vi "libdaq_counter_config.vi"(0 "error in (no error)":errorcluster, 1 "device_name":string, 2 "module_name":string, 3 "mode":T2(ring), 4 "edge":T1(ring), 5 "period":i32) -> (14 "error out":errorcluster, 15 "device_name":string, 16 "module_name":string)   [LabVIEW 2010, in "libdaqVI.lvlib"]
uses:
  libdaqVI.lvlib
  dll/daqlib.dll
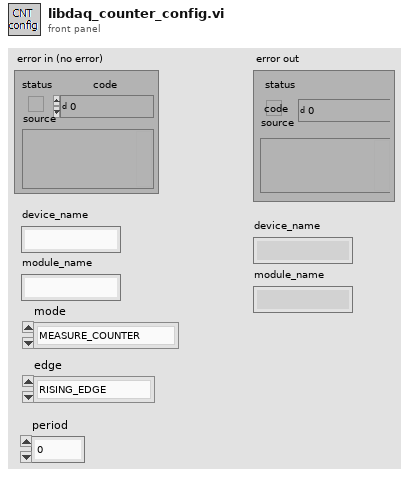
[diagram p1: front panel]
types:
  T1 = enum16{"RISING_EDGE", "FALLING_EDGE", "BOTH_EDGE"}
  T2 = enum16{"MEASURE_COUNTER", "MEASURE_PERIOD", "MEASURE_PWM"}
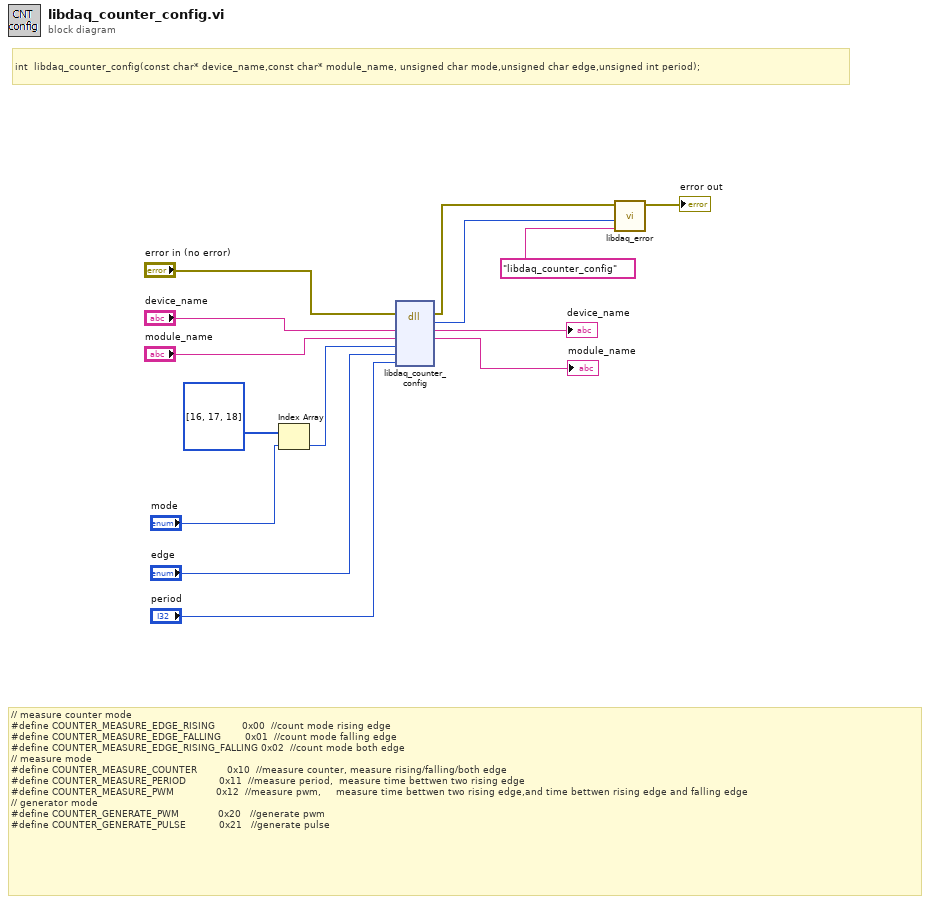
[diagram p0: block diagram]
diagram:
  # "// measure counter mode\n#define COUNTER_MEASURE_EDGE_RISING         0x00  //count mode rising edge\n#define COUNTER_MEASURE_EDGE_FALLING        0x01  //count mode falling edge\n#define COUNTER_MEASURE_EDGE_RISING_FALLING 0x02  //count mode both edge\n// measure mode\n#define COUNTER_MEASURE_COUNTER          0x10  //measure counter, measure rising/falling/both edge\n#define COUNTER_MEASURE_PERIOD           0x11  //measure period,  measure time bettwen two rising edge\n#define COUNTER_MEASURE_PWM              0x12  //measure pwm,     measure time bettwen two rising edge,and time bettwen rising edge and falling edge\n// generator mode\n#define COUNTER_GENERATE_PWM             0x20   //generate pwm\n#define COUNTER_GENERATE_PULSE           0x21   //generate pulse"
  # "int  libdaq_counter_config(const char* device_name,const char* module_name, unsigned char mode,unsigned char edge,unsigned int period);"
  n1 = Index Array(array=i32[] [16, 17, 18], index="mode") -> (element=w3:i32)
  n2 = dll-call lib="E:/Product/Example/DAQ-USB3212/Labview/labview_2010/libdaqVI/dll/daqlib.dll" fn="libdaq_counter_config"(error in="error in (no error)", "device_name"="device_name", "module_name"="module_name", "mode"=w3, "edge"="edge", "period"="period") -> (error out=w9:errorcluster, "return type"=w7:i32, "device_name"=→"device_name":string, "module_name"=→"module_name":string)  [unwired: 5 in, 1 out]
  n3 = call "libdaq_error.vi"("error source"="libdaq_counter_config", "error code"=w7, "错误输入（无错误）"=w9) -> ("错误输出"=→"error out":errorcluster)  [unwired: 8 in]
